vi "Sort Panels.vi"(7 "Sort Order":T1, 8 "error in (no error)":errorcluster, 11 "AppListPanel":refnum<class "AppListPanel.lvclass">) -> (0 "error out":errorcluster)   [LabVIEW 2020, in "PicoG-App.lvlib" / "AppListPanel.lvclass"]
uses:
  AppListPanel.lvclass
  Sort Order.ctl
  AppListPanel.lvclass/AppListPanel.ctl
  Sort By Updated.vi
  Sort By Name.vi
  <vilib>/IlluminatedG/IG OOPanel/OOPanel/ArrayManager/ArrayManager.lvclass
  <vilib>/IlluminatedG/IG OOPanel/OOPanel/Panel/Panel.lvclass
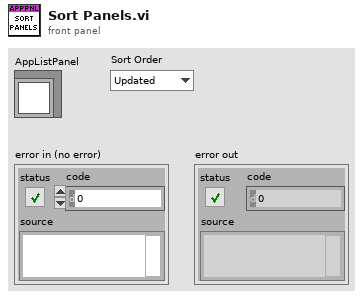
[diagram p1: front panel]
types:
  T1 = typedef "PicoG-App.lvlib/AppListPanel.lvclass/Sort Order.ctl" = enum16{"Updated", "Name"}
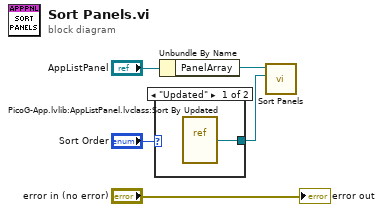
[diagram p0: block diagram]
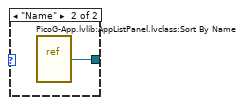
[diagram p2: hidden frame]
diagram:
  n1 = case shown="\"Updated\"" "Sort Order" {
    tunnel: [w6 w7] -> w4
    frame "Updated" {
      n2 = vi-ref "PicoG-App.lvlib:AppListPanel.lvclass:Sort By Updated.vi"() -> (w6:refnum<vi>)
    }
    frame "Name" {
      n3 = vi-ref "PicoG-App.lvlib:AppListPanel.lvclass:Sort By Name.vi"() -> (w7:refnum<vi>)
    }
  }
  n4 = Unbundle By Name("AppListPanel") -> ("PanelArray"=w2:refnum<class "ArrayManager.lvclass">)
  n5 = call <vilib>:"Sort Panels.vi"("Sort VI"=w4, "ArrayManager in"=w2) -> ()  [unwired: 8 in, 2 out]
  "error out" <- "error in (no error)"
